vi "Read All Channels.vi"(8 "error in (no error)":errorcluster, 11 "PAS":T1) -> (0 "error out":errorcluster, 3 "CAN Values":dbl[](array[numeric]))   [LabVIEW 2014]
doc: "This VI is used as to not overload the CAN boards for acquiring data. The intent is to acquire one sample/second from the NI-DAQ hardware and one sample/5 seconds from the CAN boards. At the end of every 5 second cycle, fresh values are acquired. If in the middle of the 5 second wait, the last values are used. Please note that there is no timing inside this VI, it is solely dependent on the timing of the owning VI"
uses:
  CAN Communication/PAS/Typedefs/Session Handle.ctl
  CAN Communication/PAS/PAS.lvclass
  CAN Communication/PAS/Typedefs/Pressure Sensor.ctl
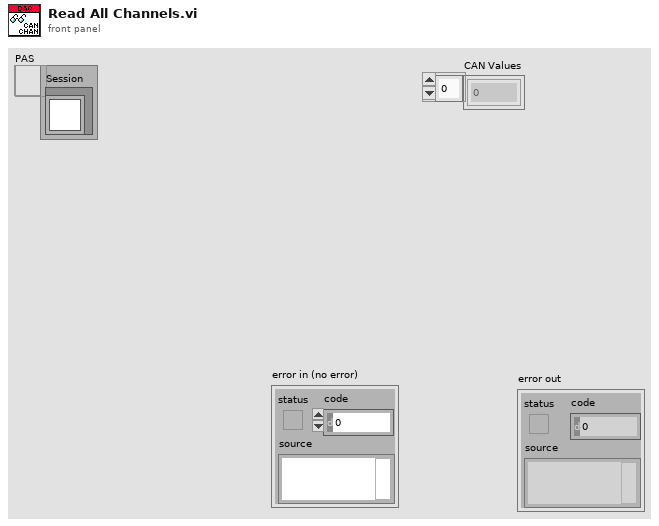
[diagram p1: front panel]
types:
  T1 = typedef "PAS.lvclass/Session Handle.ctl" = refnum<data-value>
  T2 = typedef "PAS.lvclass/Pressure Sensor.ctl" = u16
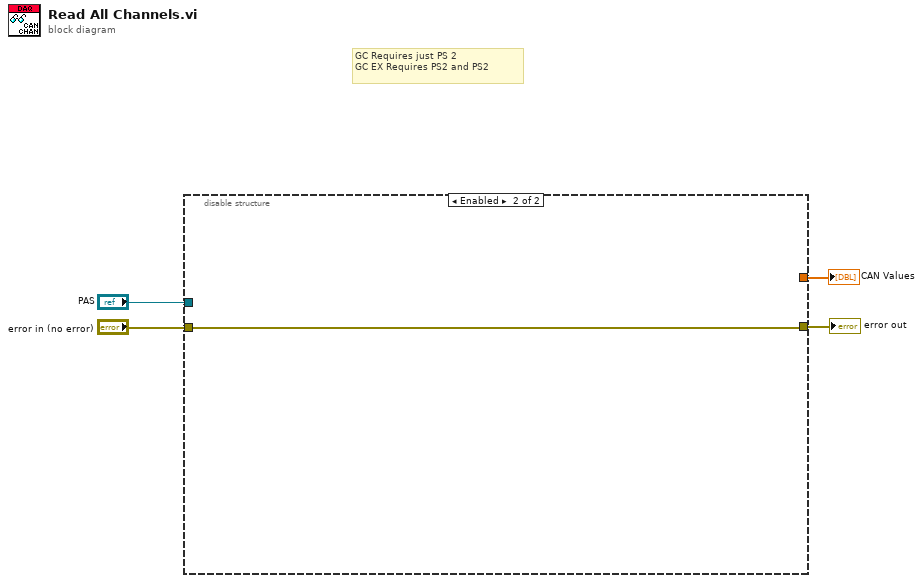
[diagram p0: block diagram]
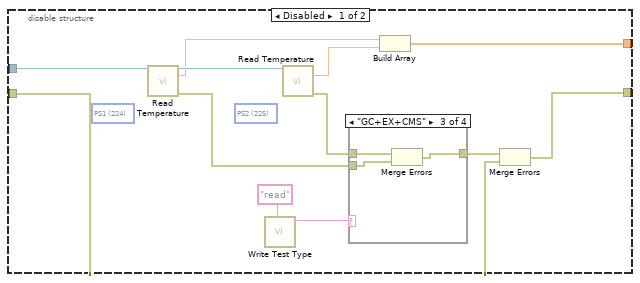
[diagram p2: hidden frame]
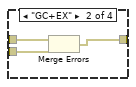
[diagram p4: hidden frame]
diagram:
  # "GC Requires just PS 2\nGC EX Requires PS2 and PS2"
  n1 = disable-structure shown="Enabled" {
    disable-tunnel: "PAS" -> [w16 _]
    disable-tunnel: [w15 _] -> w3
    disable-tunnel: "error in (no error)" -> [w7 w25]
    disable-tunnel: [w6 w25] -> w1
    frame Disabled {
      (unwired) T2 224 items=["PS1"=224, "PS2"=225] ("Pressure Sensor")
      (unwired) T2 225 items=["PS1"=224, "PS2"=225] ("Pressure Sensor")
      n2 = call "Read Temperature.vi"("Session Handle in"=w16) -> ("Session Handle out"=w13:T1, "Temperature"=w12:dbl, "error out"=w5:errorcluster)  [unwired: 12 in]
      n3 = call "Write Test Type.vi"("Command"="read") -> ("Test"=w10:string)  [unwired: 10 in]
      n4 = call "Read Temperature.vi"("Session Handle in"=w13) -> ("Temperature"=w14:dbl, "error out"=w9:errorcluster)  [unwired: 12 in, 1 out]
      n5 = case shown="\"GC+EX+CMS\"" w10 {
        tunnel: w9 -> [w17 w20 w23 w24]
        tunnel: [w17 w18 w21 w24] -> w8
        tunnel: w5 -> [_ w19 w22 _]
        frame "GC" {
        }
        frame "GC+EX" {
          n6 = Merge Errors(w20, w19) -> (w18:errorcluster)
        }
        frame "GC+EX+CMS" {
          n7 = Merge Errors(w23, w22) -> (w21:errorcluster)
        }
        frame Default {
        }
      }
      n8 = Build Array(w12, w14) -> (w15:dbl[])
      n9 = Merge Errors(w8, w7) -> (w6:errorcluster)
    }
    frame Enabled {
    }
  }
  "error out" <- w1
  "CAN Values" <- w3
